vi "Threshold.vi"(9 "Threshold Percent":dbl, 10 "Number In":dbl) -> (2 "Number Out":dbl)   [LabVIEW 2015]
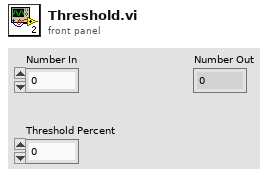
[diagram p1: front panel]
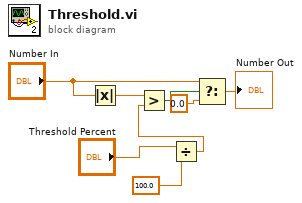
[diagram p0: block diagram]
diagram:
  n1 = Absolute Value(x="Number In") -> (abs(x)=w6:dbl)
  n2 = Divide(x="Threshold Percent", y=100.0) -> (x/y=w1:dbl)
  n3 = Greater?(x=w6, y=w1) -> (0:w5:bool)
  n4 = Select(t="Number In", s=w5, f=0.0) -> (s? t:f=→"Number Out":dbl)
